vi "lvstyx_write_path_bool.vi"(7 "Log? (T)":bool=TRUE, 8 "error in (no error)":errorcluster, 9 "boolean":bool, 10 "path":string, 11 "client ptr":u32) -> (0 "error out":errorcluster, 3 "dup client ptr":u32)   [LabVIEW 2010, in "lib1299.lvlib"]
uses:
  lib1299.lvlib
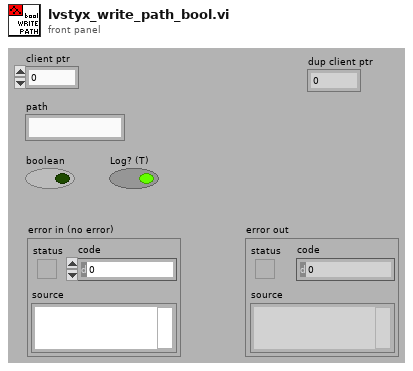
[diagram p1: front panel]
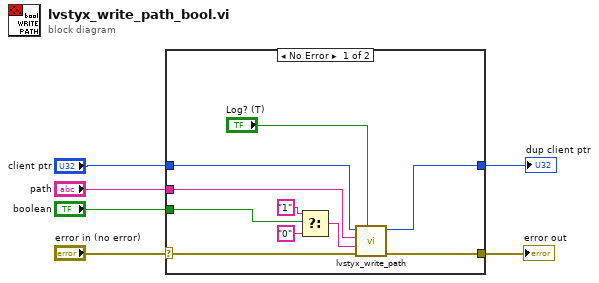
[diagram p0: block diagram]
diagram:
  n1 = case shown="No Error" "error in (no error)" {
    selector: "error in (no error)" -> [w12 w18]
    tunnel: [w13 w18] -> w6
    tunnel: "boolean" -> [w10 _]
    tunnel: "path" -> [w9 _]
    tunnel: "client ptr" -> [w8 w17]
    tunnel: [w7 w17] -> w1
    frame No Error {
      n2 = Select(t="1", s=w10, f="0") -> (s? t:f=w16:string)
      n3 = call "lvstyx_write_path.vi"("Log? (T)"="Log? (T)", "error in (no error)"=w12, "buf"=w16, "path"=w9, "client ptr"=w8) -> ("error out"=w13:errorcluster, "dup client ptr"=w7:u32)  [unwired: 4 in, 1 out]
    }
    frame Error {
    }
  }
  "error out" <- w6
  "dup client ptr" <- w1
